vi "get&set Resolution.vi"(8 "error in (no error)":errorcluster, 10 "3D Resolution":T1, 11 "VGS_VolumeDescriptor in":refnum<class "VGS_VolumeDescriptor.lvclass">) -> (0 "error out":errorcluster, 2 "3D Size":T1, 3 "VGS_VolumeDescriptor out":refnum<class "VGS_VolumeDescriptor.lvclass">)   [LabVIEW 2022 SP3, in "LV_VGS.lvlib" / "VGS_VolumeDescriptor.lvclass"]
uses:
  VGS_VolumeDescriptor.lvclass
  typedefs/3D Resolution (SGL).ctl
  VGS_VolumeDescriptor.lvclass/VGS_VolumeDescriptor.ctl
  C:/Users/Andrey/Desktop/hajo/LV_VGS/vgs_project.dll
  vgs_project.dll
  LV_VGS.lvlib
panel:
  in  "Get/Set? (Set)":bool=TRUE
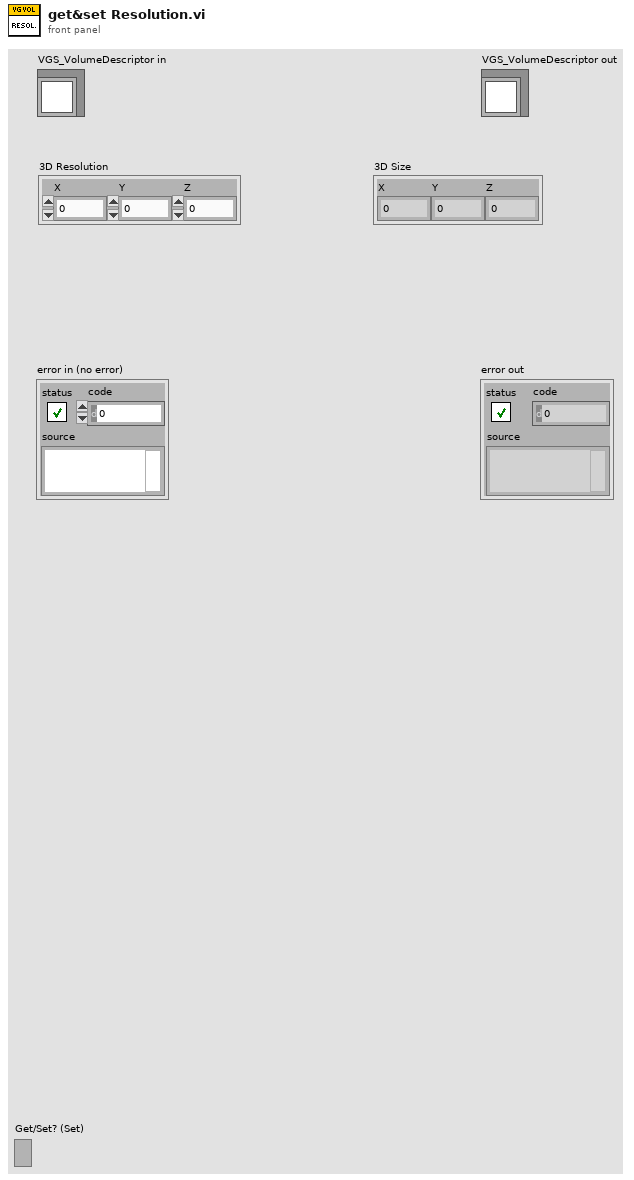
[diagram p1: front panel]
types:
  T1 = typedef "LV_VGS.lvlib/3D Resolution (SGL).ctl" = cluster{"X":sgl, "Y":sgl, "Z":sgl}
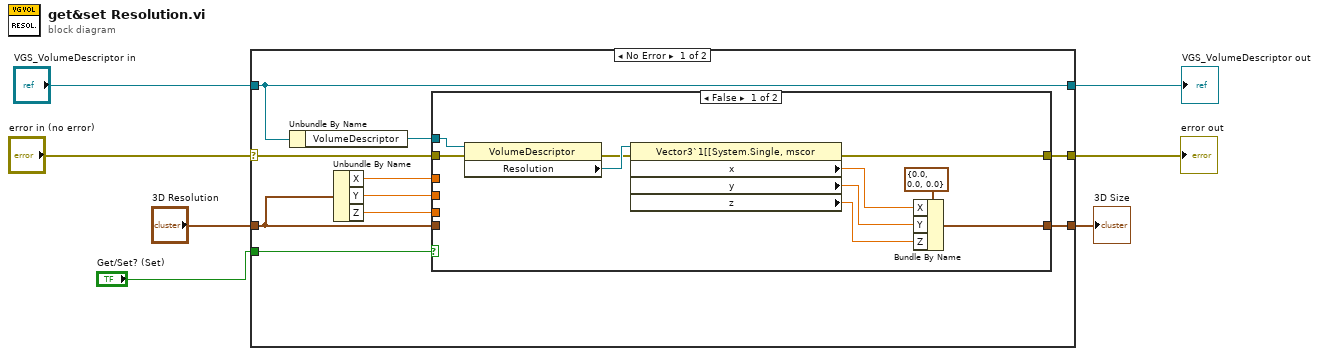
[diagram p0: block diagram]
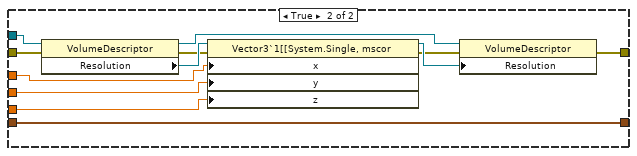
[diagram p2: hidden frame]
diagram:
  n1 = case shown="No Error" "error in (no error)" {
    selector: "error in (no error)" -> [w15 w42]
    tunnel: [w14 w42] -> w1
    tunnel: [w17 w41] -> w2
    tunnel: "VGS_VolumeDescriptor in" -> [w17 w41]
    tunnel: "Get/Set? (Set)" -> [w13 _]
    tunnel: [w12 w40] -> w5
    tunnel: "3D Resolution" -> [w8 w40]
    frame No Error {
      n2 = Unbundle By Name(w17) -> ("VolumeDescriptor"=w16:refnum<k24>)
      n3 = Unbundle By Name(w8) -> ("X"=w11:sgl, "Y"=w10:sgl, "Z"=w9:sgl)
      n4 = case shown="False" w13 {
        tunnel: w16 -> [w27 w33]
        tunnel: w15 -> [w26 w31]
        tunnel: [w18 w34] -> w14
        tunnel: w8 -> [_ w39]
        tunnel: [w20 w39] -> w12
        tunnel: w11 -> [_ w28]
        tunnel: w10 -> [_ w38]
        tunnel: w9 -> [_ w37]
        frame False {
          n5 = property class="VolumeDescriptor"(reference=w27, error in=w26) -> (error out=w19:errorcluster, "Resolution"=w25:refnum<k24>)  [unwired: 1 out]
          n6 = property class="Vector3`1[[System.Single, mscor"(reference=w25, error in=w19) -> (error out=w18:errorcluster, "x"=w23:sgl, "y"=w22:sgl, "z"=w21:sgl)  [unwired: 1 out]
          n7 = Bundle By Name(cluster=T1 {"X"=0.0, "Y"=0.0, "Z"=0.0} ("3D Size"), "X"=w23, "Y"=w22, "Z"=w21) -> (w20:T1)
        }
        frame True {
          n8 = property class="VolumeDescriptor"(reference=w33, error in=w31) -> (reference out=w29:refnum<k24>, error out=w30:errorcluster, "Resolution"=w32:refnum<k24>)
          n9 = property class="Vector3`1[[System.Single, mscor"(reference=w32, error in=w30, "x"=w28, "y"=w38, "z"=w37) -> (reference out=w36:refnum<k24>, error out=w35:errorcluster)
          n10 = property class="VolumeDescriptor"(reference=w29, error in=w35, "Resolution"=w36) -> (error out=w34:errorcluster)  [unwired: 1 out]
        }
      }
    }
    frame Error {
    }
  }
  "error out" <- w1
  "VGS_VolumeDescriptor out" <- w2
  "3D Size" <- w5
